vi "FGV - Condition.vi"(7 "Action":T1=enum."R", 8 "error in (no error)":errorcluster, 11 "array in":string[][](array[string])) -> (0 "error out":errorcluster, 3 "array out":string[][](array[string]))   [LabVIEW 2018]
uses:
  CTL/FGV - R-W.ctl
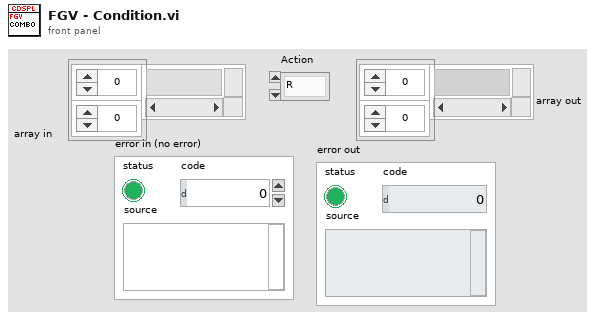
[diagram p1: front panel]
types:
  T1 = typedef "FGV - R-W.ctl" = enum16{"W", "R"}
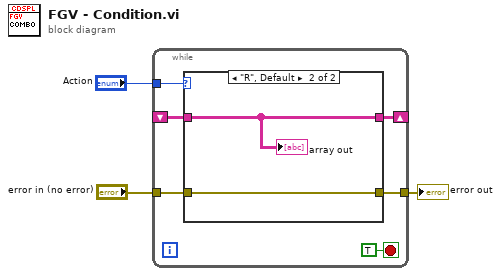
[diagram p0: block diagram]
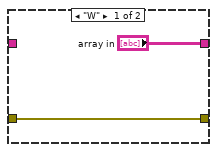
[diagram p2: hidden frame]
diagram:
  n1 = while {
    tunnel: "Action" -> [w9]
    tunnel: "error in (no error)" -> [w8]
    tunnel: [w7] -> w1
    shift-right: [w6] -> _
    shift-left: _ -> [w5]
    stop <- TRUE stop-if-true
    n2 = case shown="\"R\", Default" w9 {
      tunnel: [w11 w13] -> w7
      tunnel: w8 -> [w11 w13]
      tunnel: ["array in" w12] -> w6
      tunnel: w5 -> [_ w12]
      frame "W" {
      }
      frame "R", Default {
        "array out" <- w12
      }
    }
  }
  "error out" <- w1
